vi "CmdConsole.Get StdOut, StdError, and Rtn Code.vi"(8 "error in (no error)":errorcluster, 11 "CmdConsole in":refnum<class "CmdConsole.lvclass">) -> (0 "error out":errorcluster, 1 "StdErr":string, 2 "StdOut":string, 3 "CmdConsole out":refnum<class "CmdConsole.lvclass">, 4 "Rtn Code":i32)   [LabVIEW 2018, in "CmdConsole.lvclass"]
uses:
  CmdConsole.lvclass
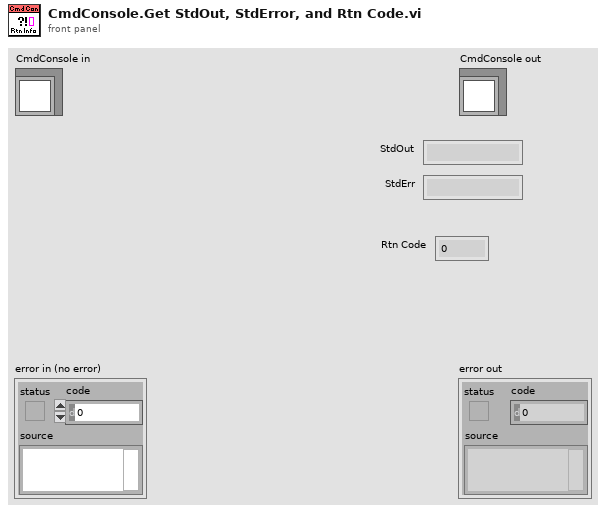
[diagram p1: front panel]
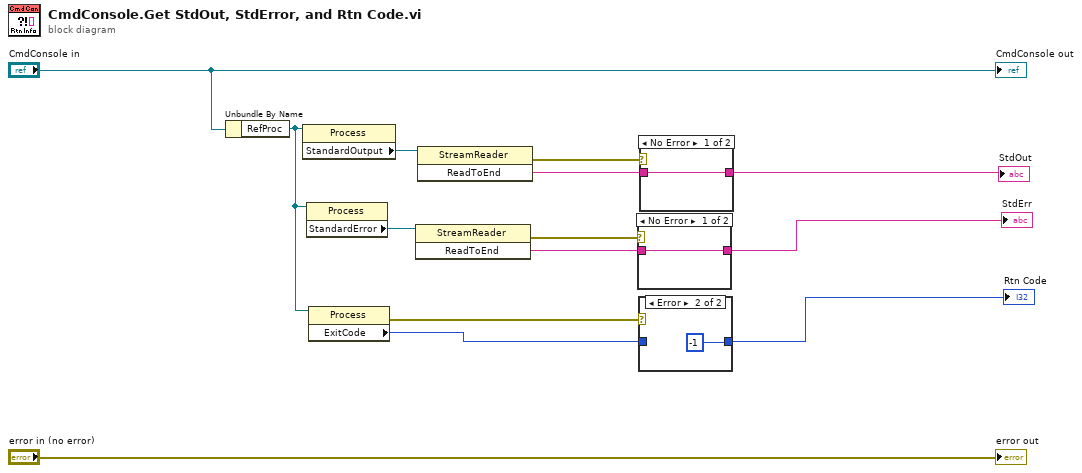
[diagram p0: block diagram]
diagram:
  n1 = Unbundle By Name("CmdConsole in") -> ("RefProc"=w4:refnum<k24>)
  n2 = property class="Process"(reference=w4) -> ("StandardOutput"=w10:refnum<k24>)  [unwired: 1 in, 2 out]
  n3 = property class="Process"(reference=w4) -> ("StandardError"=w5:refnum<k24>)  [unwired: 1 in, 2 out]
  n4 = property class="Process"(reference=w4) -> (error out=w3:errorcluster, "ExitCode"=w2:i32)  [unwired: 1 in, 1 out]
  n5 = invoke class="StreamReader" method="ReadToEnd"(reference=w5) -> (error out=w6:errorcluster, "ReadToEnd"=w7:string)  [unwired: 2 in, 1 out]
  n6 = invoke class="StreamReader" method="ReadToEnd"(reference=w10) -> (error out=w9:errorcluster, "ReadToEnd"=w8:string)  [unwired: 2 in, 1 out]
  n7 = case shown="No Error" w6 {
    tunnel: w7 -> [w15 _]
    tunnel: [w15 _] -> w12
    frame No Error {
    }
    frame Error {
    }
  }
  "StdErr" <- w12
  n8 = case shown="Error" w3 {
    tunnel: [w16 -1] -> w11
    tunnel: w2 -> [w16 _]
    frame No Error {
    }
    frame Error {
    }
  }
  "Rtn Code" <- w11
  n9 = case shown="No Error" w9 {
    tunnel: w8 -> [w18 _]
    tunnel: [w18 _] -> w13
    frame No Error {
    }
    frame Error {
    }
  }
  "StdOut" <- w13
  "error out" <- "error in (no error)"
  "CmdConsole out" <- "CmdConsole in"
